vi "Get Adjacency.vi"(8 "error in (no error)":errorcluster, 11 "Maze in":refnum<class "Maze.lvclass">) -> (0 "error out":errorcluster, 2 "Adjacency":T1[][](array[typedef]), 3 "Maze out":refnum<class "Maze.lvclass">)   [LabVIEW 2020, in "Maze.lvlib" / "Maze.lvclass"]
uses:
  Maze.lvclass
  Adjacency.ctl
  Maze.lvclass/Maze.ctl
  Maze.lvlib
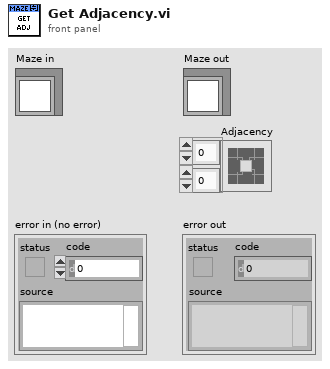
[diagram p1: front panel]
types:
  T1 = typedef "Maze.lvlib/Adjacency.ctl" = cluster{"E":bool, "N":bool, "W":bool, "S":bool, "Goal":bool, "Start":bool}
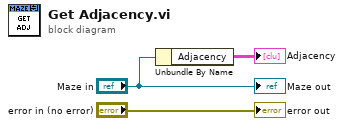
[diagram p0: block diagram]
diagram:
  n1 = Unbundle By Name("Maze in") -> ("Adjacency"=→"Adjacency":T1[][])
  "error out" <- "error in (no error)"
  "Maze out" <- "Maze in"
